vi "test-PID-input-output.vi"() -> ()   [LabVIEW 2019]
uses:
  <vilib>/Rock Robotics/WPI/ThirdParty/JAS_Junk/TrajLib/PIDController_NewPeriod.vi
  <vilib>/Rock Robotics/WPI/ThirdParty/JAS_Junk/TrajLib/PIDController_SetSetpoint.vi
  <vilib>/Rock Robotics/WPI/ThirdParty/JAS_Junk/TrajLib/PIDController_Calculate_PV.vi
  <vilib>/Rock Robotics/WPI/ThirdParty/JAS_Junk/TrajLib/PIDController_SetInputRange.vi
  <vilib>/Rock Robotics/SystemInterfaces/NetworkCommunication/NetComm_UsageReport_report.vi
  <vilib>/Rock Robotics/WPI/ThirdParty/JAS_Junk/TrajLib/PIDController_GetContinuousError.vi
  <vilib>/Rock Robotics/WPI/ThirdParty/JAS_Junk/TrajLib/Util_LibraryGlobals.vi
  <vilib>/Rock Robotics/WPI/ThirdParty/JAS_Junk/TrajLib/Trajectory_Library.lvlib
panel:
  out "T3 -- Output =":dbl
  out "T2 -- Output  = -0.01":dbl
  out "T1 -- Output  = -0.1":dbl
  out "T0 -- Output < 0":dbl
  # "PID Input Output"
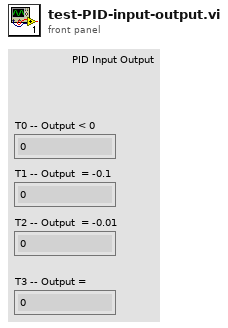
[diagram p1: front panel]
types:
  T1 = typedef "Trajectory_Library.lvlib/PID_CONTROLLER.ctl" = cluster{"Kp":dbl, "Ki":dbl, "Kd":dbl, "Period":dbl, "Max_Integral":dbl, "Min_Integral":dbl, "Max_Input":dbl, "Min_Input":dbl, "Input_Range":dbl, "Continuous":bool, "PositionError":dbl, "VelocityError":dbl, "PrevError":dbl, "TotalError":dbl, "PositionTolerance":dbl, "VelocityTolerance":dbl, "SetPoint":dbl, "Kf":dbl, "Prev_Deriv":dbl, "Prev_Deriv 2":dbl, "DerivativeFilter":bool, "Min_Output":dbl, "Max_Output":dbl, "Prev_F_P":dbl, "Prev_F_P_2":dbl, "AntiWindupActive":bool}
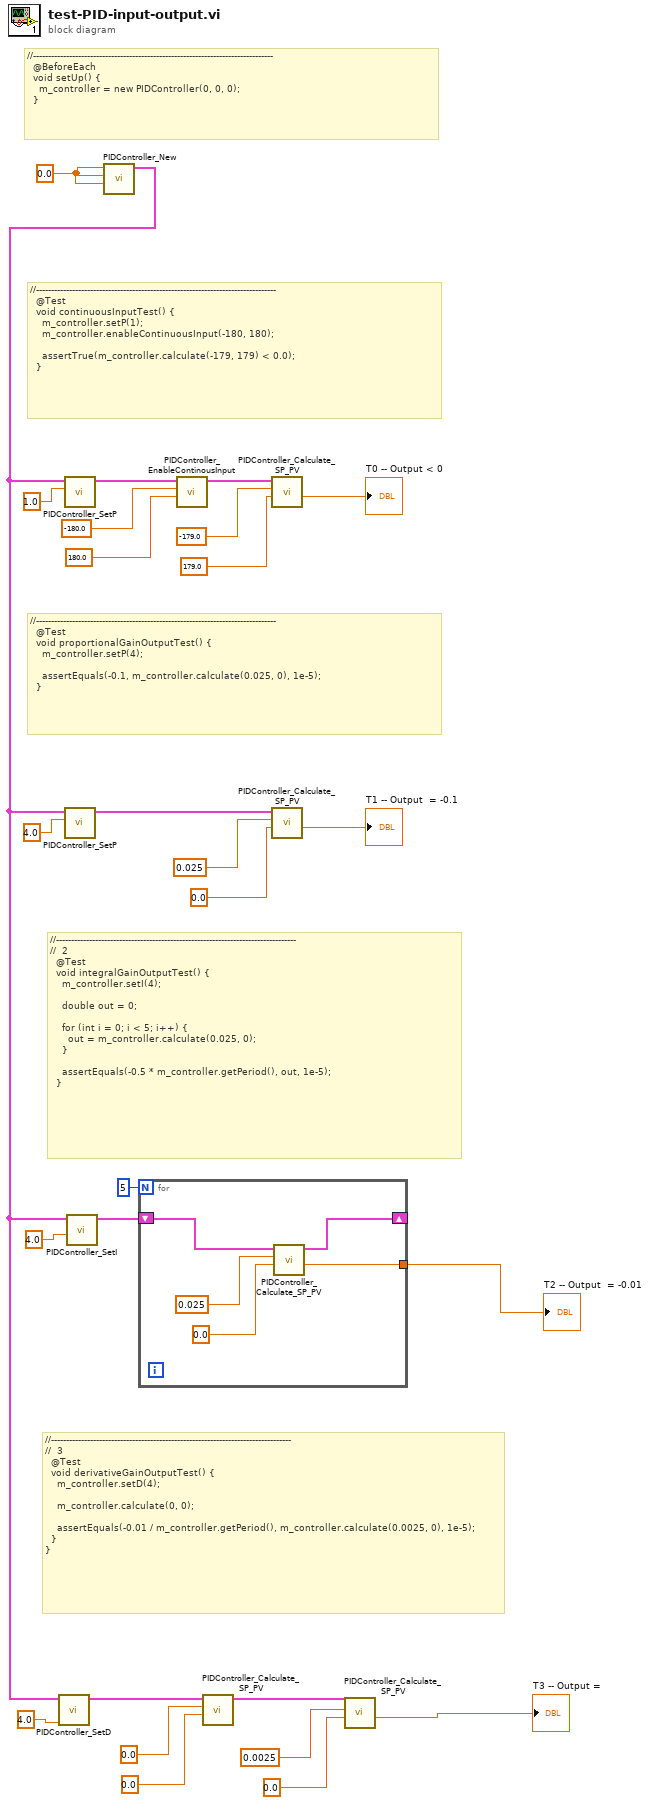
[diagram p0: block diagram]
diagram:
  w27 = 0.0 ("Kp")
  # "//--------------------------------------------------------------------------------\n//  3\n  @Test\n  void derivativeGainOutputTest() {\n    m_controller.setD(4);\n\n    m_controller.calculate(0, 0);\n\n    assertEquals(-0.01 / m_controller.getPeriod(), m_controller.calculate(0.0025, 0), 1e-5);\n  }\n}"
  # "//--------------------------------------------------------------------------------\n//  2\n  @Test\n  void integralGainOutputTest() {\n    m_controller.setI(4);\n\n    double out = 0;\n\n    for (int i = 0; i < 5; i++) {\n      out = m_controller.calculate(0.025, 0);\n    }\n\n    assertEquals(-0.5 * m_controller.getPeriod(), out, 1e-5);\n  }"
  # "//--------------------------------------------------------------------------------\n  @Test\n  void proportionalGainOutputTest() {\n    m_controller.setP(4);\n\n    assertEquals(-0.1, m_controller.calculate(0.025, 0), 1e-5);\n  }"
  # "//--------------------------------------------------------------------------------\n  @BeforeEach\n  void setUp() {\n    m_controller = new PIDController(0, 0, 0);\n  }"
  # "//--------------------------------------------------------------------------------\n  @Test\n  void continuousInputTest() {\n    m_controller.setP(1);\n    m_controller.enableContinuousInput(-180, 180);\n\n    assertTrue(m_controller.calculate(-179, 179) < 0.0);\n  }"
  n1 = call <vilib>:"PIDController_New.vi"("Kd"=w27, "Ki"=w27, "Kp"=w27) -> ("PID_CONTROLLER"=w5:T1)  [unwired: 8 in]
  n2 = call <vilib>:"PIDController_SetD.vi"("Kd"=4.0 ("Kp"), "in PID_CONTROLLER"=w5) -> ("out PID_CONTROLLER"=w8:T1)  [unwired: 9 in]
  n3 = call <vilib>:"PIDController_SetP.vi"("Kp"=1.0, "in PID_CONTROLLER"=w5) -> ("out PID_CONTROLLER"=w25:T1)  [unwired: 9 in]
  n4 = call <vilib>:"PIDController_SetP.vi"("Kp"=4.0, "in PID_CONTROLLER"=w5) -> ("out PID_CONTROLLER"=w14:T1)  [unwired: 9 in]
  n5 = call <vilib>:"PIDController_SetI.vi"("Ki"=4.0 ("Kp"), "in PID_CONTROLLER"=w5) -> ("out PID_CONTROLLER"=w11:T1)  [unwired: 9 in]
  n6 = for {
    N: 5 -> [_]
    tunnel: [w30] -> w12
    shift-right: [w28] -> _
    shift-left: w11 -> [w29]
    n7 = call <vilib>:"PIDController_Calculate_SP_PV.vi"("SP-SetPoint"=0.0, "PV-Measurement"=0.025, "in PID_CONTROLLER"=w29) -> ("CO-ControlOutput"=w30:dbl, "out PID_CONTROLLER"=w28:T1)  [unwired: 7 in]
  }
  "T2 -- Output  = -0.01" <- w12
  n8 = call <vilib>:"PIDController_EnableContinousInput.vi"("MaxInput"=180.0, "MinInput"=-180.0, "in PID_CONTROLLER"=w25) -> ("out PID_CONTROLLER"=w22:T1)  [unwired: 8 in]
  n9 = call <vilib>:"PIDController_Calculate_SP_PV.vi"("SP-SetPoint"=0.0, "PV-Measurement"=0.0, "in PID_CONTROLLER"=w8) -> ("out PID_CONTROLLER"=w2:T1)  [unwired: 7 in, 1 out]
  n10 = call <vilib>:"PIDController_Calculate_SP_PV.vi"("SP-SetPoint"=179.0, "PV-Measurement"=-179.0, "in PID_CONTROLLER"=w22) -> ("CO-ControlOutput"=→"T0 -- Output < 0":dbl)  [unwired: 7 in, 1 out]
  n11 = call <vilib>:"PIDController_Calculate_SP_PV.vi"("SP-SetPoint"=0.0, "PV-Measurement"=0.025, "in PID_CONTROLLER"=w14) -> ("CO-ControlOutput"=→"T1 -- Output  = -0.1":dbl)  [unwired: 7 in, 1 out]
  n12 = call <vilib>:"PIDController_Calculate_SP_PV.vi"("SP-SetPoint"=0.0, "PV-Measurement"=0.0025, "in PID_CONTROLLER"=w2) -> ("CO-ControlOutput"=→"T3 -- Output =":dbl)  [unwired: 7 in, 1 out]
